vi "SMO.Dictionary.GetValues.vi"(6 "timeout (10ms)":i32=10, 8 "error in (no error)":errorcluster, 10 "Keys (empty: All)":string[](array[string]), 11 "SMO.Dictionary":refnum<class "SMO.Dictionary.lvclass">) -> (0 "error out":errorcluster, 1 "Values":variant[](array[variant]), 2 "Keys out":string[](array[string]), 3 "SMO.Dictionary out":refnum<class "SMO.Dictionary.lvclass">, 4 "timed out?":bool)   [LabVIEW 2013, in "SMO.Dictionary.lvlib" / "SMO.Dictionary.lvclass"]
doc: "---------------------------------------------------------------\nJKI State Machine Objects™\nhttp://jki.net/state-machine-objects/\nCopyright (C) 2005-2015, JKI <info@jki.net>\nALL RIGHTS RESERVEDJKI State Machine Objects (SMO) 1.0.0.4\nJKI - JKI\nCopyright (c) 2015, JKI"
uses:
  SMO.Dictionary.lvclass
  Typedefs/PrivateEvents--SMO.Dictionary.GetMultipleValues.ctl
  Typedefs/PrivateEvents--SMO.Dictionary.KeyValue-Pair Array.ctl
  <vilib>/JKI/JKI SMO/SMO/SMO.lvclass
panel:
  # "For instructions on how to use the JKI State Machine Objects, examples and video tutorials, visit:\nhttp://jki.net/state-machine-objects/\n\nJKI State Machine Objects™\nhttp://jki.net/state-machine-objects/\nCopyright (C) 2005-2015, JKI <info@jki.net>\nALL RIGHTS RESERVED"
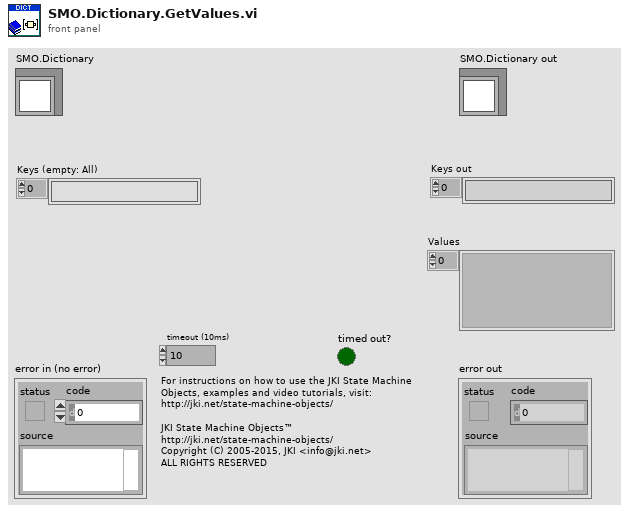
[diagram p1: front panel]
types:
  T1 = typedef "SMO.lvclass/SMOState --Enum.ctl" = enum16{"unknown", "Created", "Started", "Stopped"}
  T2 = typedef "SMO.Dictionary.lvlib/SMO.Dictionary.lvclass/PrivateEvents--SMO.Dictionary.KeyValue-Pair Array.ctl" = cluster{"Keys":string[], "Values":variant[]}
  T3 = typedef "SMO.Dictionary.lvlib/SMO.Dictionary.lvclass/PrivateEvents--SMO.Dictionary.GetMultipleValues.ctl" = cluster{"Keys":string[], "response":refnum<notifier>}
  T4 = typedef "SMO.Dictionary.lvlib/SMO.Dictionary.lvclass/PrivateEvents--Cluster.ctl" = cluster{"Update":refnum<user-event>, "Clear Dictionary":refnum<user-event>, "Delete":refnum<user-event>, "Get":refnum<user-event>, "GetMultiple":refnum<user-event>}
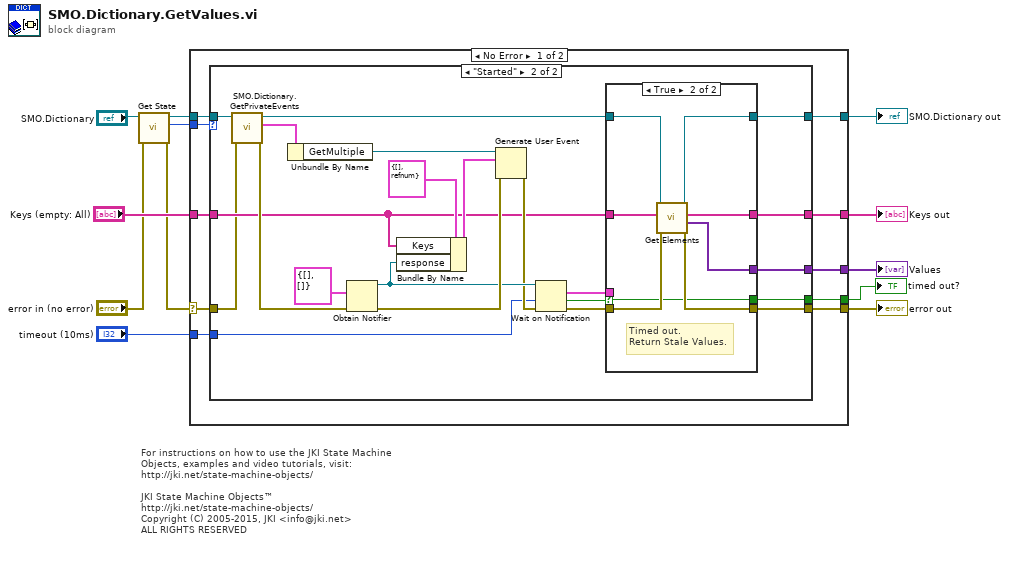
[diagram p0: block diagram]
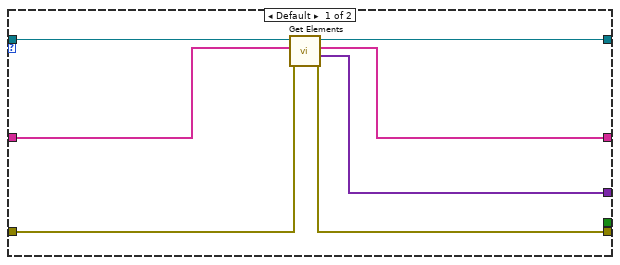
[diagram p2: hidden frame]
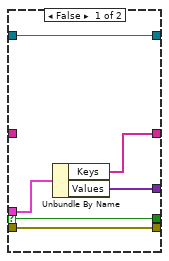
[diagram p3: hidden frame]
diagram:
  # "For instructions on how to use the JKI State Machine Objects, examples and video tutorials, visit:\nhttp://jki.net/state-machine-objects/\n\nJKI State Machine Objects™\nhttp://jki.net/state-machine-objects/\nCopyright (C) 2005-2015, JKI <info@jki.net>\nALL RIGHTS RESERVED"
  n1 = call <vilib>:"Get State.vi"("error in (no error)"="error in (no error)", "SMO"="SMO.Dictionary") -> ("error out"=w2:errorcluster, "SMO State"=w1:T1, "SMO out"=w4:refnum<class "SMO.Dictionary.lvclass">)  [unwired: 7 in]
  n2 = case shown="No Error" w2 {
    selector: w2 -> [w14 w68]
    tunnel: "timeout (10ms)" -> [w22 _]
    tunnel: "Keys (empty: All)" -> [w21 w67]
    tunnel: [w20 w66] -> w10
    tunnel: [w19 w68] -> w9
    tunnel: [w18 _] -> w8
    tunnel: [w17 w67] -> w7
    tunnel: [w16 _] -> w6
    tunnel: w4 -> [w15 w66]
    tunnel: w1 -> [w13 _]
    frame No Error {
      n3 = case shown="\"Started\"" w13 {
        tunnel: w22 -> [_ w42]
        tunnel: w21 -> [w28 w41]
        tunnel: [w23 w39] -> w20
        tunnel: [w26 w37] -> w19
        tunnel: [_ w34] -> w18
        tunnel: [w24 w33] -> w17
        tunnel: [w25 w32] -> w16
        tunnel: w15 -> [w29 w31]
        tunnel: w14 -> [w27 w30]
        frame Default {
          n4 = call-dynamic "Get Elements.vi"("error in (no error)"=w27, "Keys (empty: All)"=w28, "SMO.Dictionary in"=w29) -> ("error out"=w26:errorcluster, "Values"=w25:variant[], "Keys out"=w24:string[], "SMO.Dictionary out"=w23:refnum<class "SMO.Dictionary.lvclass">)  [unwired: 5 in]
        }
        frame "Started" {
          n5 = call "SMO.Dictionary.GetPrivateEvents.vi"("error in (no error)"=w30, "SMO.Dictionary"=w31) -> ("error out"=w51:errorcluster, "Private Events"=w50:T4, "SMO.Dictionary out"=w40:refnum<class "SMO.Dictionary.lvclass">)  [unwired: 7 in]
          n6 = Unbundle By Name(w50) -> ("GetMultiple"=w45:refnum<user-event>)
          n7 = Obtain Notifier(notification data type=T2 {"Keys"=[], "Values"=[]} ("KeyValue Pairs"), error in (no error)=w51) -> (notifier out=w47:refnum<notifier>, error out=w48:errorcluster)  [unwired: 2 in, 1 out]
          n8 = Bundle By Name(cluster=T3 {"Keys"=[], "response"=refnum} ("GetMultiple"), "Keys"=w41, "response"=w47) -> (w49:T3)
          n9 = Generate User Event(user event=w45, event data cluster=w49, error in=w48) -> (error out=w46:errorcluster)  [unwired: 1 in, 1 out]
          n10 = Wait on Notification(notifier=w47, timeout in ms (-1)=w42, error in (no error)=w46) -> (notification=w35:T2, timed out?=w36:bool, error out=w38:errorcluster)  [unwired: 1 in, 1 out]
          n11 = case shown="True" w36 {
            selector: w36 -> [w55 w58]
            tunnel: w41 -> [_ w65]
            tunnel: w40 -> [w57 w64]
            tunnel: [w57 w63] -> w39
            tunnel: w38 -> [w56 w62]
            tunnel: [w56 w61] -> w37
            tunnel: w35 -> [w54 _]
            tunnel: [w55 w58] -> w34
            tunnel: [w53 w60] -> w33
            tunnel: [w52 w59] -> w32
            frame False {
              n12 = Unbundle By Name(w54) -> ("Keys"=w53:string[], "Values"=w52:variant[])
            }
            frame True {
              # "Timed out.\nReturn Stale Values."
              n13 = call-dynamic "Get Elements.vi"("error in (no error)"=w62, "Keys (empty: All)"=w65, "SMO.Dictionary in"=w64) -> ("error out"=w61:errorcluster, "Values"=w59:variant[], "Keys out"=w60:string[], "SMO.Dictionary out"=w63:refnum<class "SMO.Dictionary.lvclass">)  [unwired: 5 in]
            }
          }
        }
      }
    }
    frame Error {
    }
  }
  "error out" <- w9
  "SMO.Dictionary out" <- w10
  "Values" <- w6
  "Keys out" <- w7
  "timed out?" <- w8
